vi "Socket.vi"(7 "path override":path, 8 "error in (no error)":errorcluster, 10 "Socket Type":T1=enum."Request", 11 "ctx in":u64) -> (0 "error out":errorcluster, 2 "s_":u64, 3 "ctx out":u64)   [LabVIEW 2025, in "libzmq-v143-mt-4_3_6.lvlib"]
doc: "ZMQ_EXPORT void *zmq_socket (void *, int type_);"
uses:
  libzmq-v143-mt-4_3_6.lvlib
  ctls/SocketType.ctl
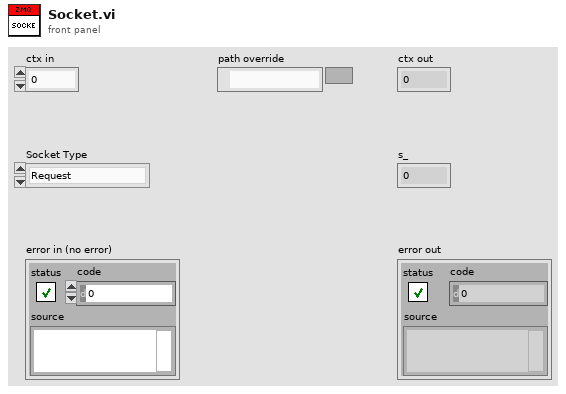
[diagram p1: front panel]
types:
  T1 = typedef "libzmq-v143-mt-4_3_6.lvlib/SocketType.ctl" = enum16{"Pair", "Pub", "Sub", "Request", "Reply", "Dealer", "Router", "Pull", "Push", "XPub", "XSub"}
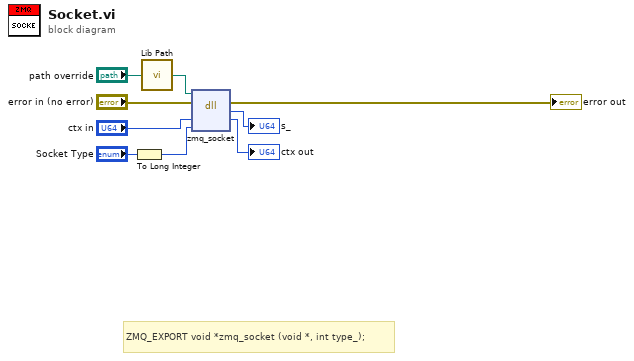
[diagram p0: block diagram]
diagram:
  # "ZMQ_EXPORT void *zmq_socket (void *, int type_);"
  n1 = To Long Integer(number="Socket Type") -> (32bit integer=w4:i32)
  n2 = call "Lib Path.vi"("path override"="path override") -> ("lib path"=w2:path)
  n3 = dll-call lib="home/james/Documents/ZeroMQ_LV/libzmq-v143-mt-4_3_6/libzmq.so" fn="zmq_socket"(path in=w2, error in="error in (no error)", "ctx"="ctx in", "type_"=w4) -> (error out=→"error out":errorcluster, "return type"=→"s_":u64, "ctx"=→"ctx out":u64)  [unwired: 2 in, 1 out]
